vi "MockFAILC1.vi"(11 "MockFAILC1Settings":T1={"ModbusTxDataFIFO"="ModbusSubnetATxDataFIFO", "Code17Memory"="MockFAILC1Code17", "BufferUpdateFIFO"="MockFAILC1Command", "ModbusRxDataFIFO"="ModbusSubnetARxDataFIFO", "Code18Memory"="MockFAILC1Code18", "Code65Memory"="MockFAILC1Code65", "Code66Memory"="MockFAILC1Code66", "Code67Memory"="MockFAILC1Code67", "Code72Memory"="MockFAILC1Code72", "Code80Memory"="MockFAILC1Code80", "Code110Memory"="MockFAILC1Code110", "CRCDataFIFO"="MockFAILC1CRCDataFIFO", "CRCCalculateFIFO"="MockFAILC1CRCCalculateFIFO", "CRCFIFO"="MockFAILC1CRCFIFO"}) -> ()   [LabVIEW 2016, in "FPGAMockFAILC.lvlib"]
uses:
  FPGAMockFAILC.lvlib
  Common_FPGA_Modbus/FPGAModbus.lvlib
  Common_FPGA_Modbus/DataTypes/ModbusCRCSettings.ctl
  DataTypes/MockFAILC1Settings.ctl
panel:
  in  "ModbusCRCSettings":T2={"DataFIFO"="MockFAILC1CRCDataFIFO", "CalculateFIFO"="MockFAILC1CRCCalculateFIFO", "OutputFIFO"="MockFAILC1CRCFIFO"}
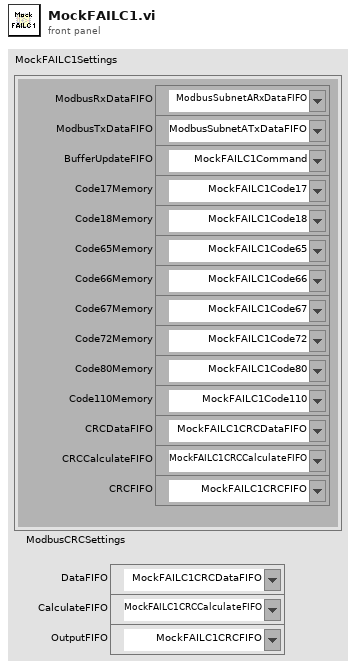
[diagram p1: front panel]
types:
  T1 = typedef "FPGAMockFAILC.lvlib/MockFAILC1Settings.ctl" = cluster{"ModbusTxDataFIFO":refnum<k21>, "Code17Memory":refnum<k21>, "BufferUpdateFIFO":refnum<k21>, "ModbusRxDataFIFO":refnum<k21>, "Code18Memory":refnum<k21>, "Code65Memory":refnum<k21>, "Code66Memory":refnum<k21>, "Code67Memory":refnum<k21>, "Code72Memory":refnum<k21>, "Code80Memory":refnum<k21>, "Code110Memory":refnum<k21>, "CRCDataFIFO":refnum<k21>, "CRCCalculateFIFO":refnum<k21>, "CRCFIFO":refnum<k21>}
  T2 = typedef "FPGAModbus.lvlib/ModbusCRCSettings.ctl" = cluster{"DataFIFO":refnum<k21>, "CalculateFIFO":refnum<k21>, "OutputFIFO":refnum<k21>}
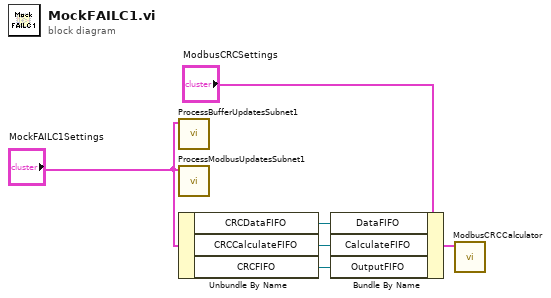
[diagram p0: block diagram]
diagram:
  n1 = call "ProcessBufferUpdatesSubnet1.vi"("MockFAILC1Settings"="MockFAILC1Settings") -> ()  [unwired: 11 in]
  n2 = call "ProcessModbusUpdatesSubnet1.vi"("MockFAILC1Settings"="MockFAILC1Settings") -> ()  [unwired: 11 in]
  n3 = Unbundle By Name("MockFAILC1Settings") -> ("CRCDataFIFO"=w5:refnum<k21>, "CRCCalculateFIFO"=w4:refnum<k21>, "CRCFIFO"=w3:refnum<k21>)
  n4 = Bundle By Name(cluster="ModbusCRCSettings", "DataFIFO"=w5, "CalculateFIFO"=w4, "OutputFIFO"=w3) -> (w2:T2)
  n5 = call "ModbusCRCCalculator.vi"("ModbusCRCSettings"=w2) -> ()  [unwired: 11 in]
